vi "Get Mapped Memory Infomation.vi"(1 "Mapped Memory Access Image ARGB in":refnum<class "Mapped Memory Access Image ARGB.lvclass">) -> (0 "Raw Memory Information":T1)   [LabVIEW 2020, in "image.lvlib" / "Mapped Memory Access Image ARGB.lvclass"]
doc: "Get the mapped memory information required for direct read/write access."
uses:
  Mapped Memory Access Image ARGB.lvclass
  Raw Memory Information.ctl
  Raw Memory Information Dimension.ctl
  Mapped Memory Access Image ARGB.lvclass/Mapped Memory Access Image ARGB.ctl
  image.lvlib
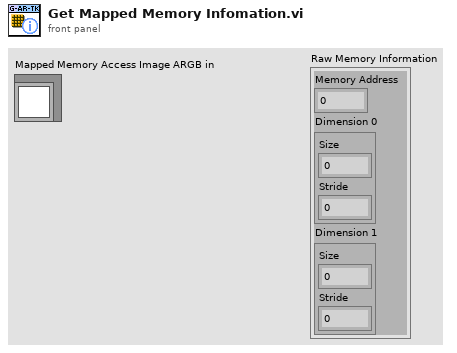
[diagram p1: front panel]
types:
  T1 = typedef "image.lvlib/Raw Memory Information.ctl" = cluster{"Memory Address":u64, "Dimension 0":T2, "Dimension 1":T2}
  T2 = typedef "image.lvlib/Raw Memory Information Dimension.ctl" = cluster{"Size":u16, "Stride":u32}
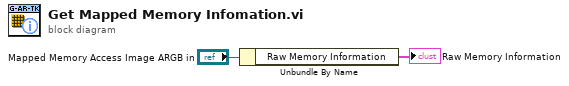
[diagram p0: block diagram]
diagram:
  n1 = Unbundle By Name("Mapped Memory Access Image ARGB in") -> ("Raw Memory Information"=→"Raw Memory Information":T1)
